vi "Projekt_KSP_main.vi"() -> ()   [LabVIEW 2020]
uses:
  <vilib>/sound2/lvsound2.llb/Sampling Mode.ctl
  <vilib>/sound2/lvsound2.llb/Sound Data Format.ctl
  <vilib>/sound2/lvsound2.llb/Sound Output Set Volume (Single).vi
  <vilib>/Utility/inputDevices.llb/keyboardAcquire.vi
  <vilib>/sound2/lvsound2.llb/Sound Output Write (DBL Single).vi
  <vilib>/Utility/inputDevices.llb/closeKeyboard.vi
  <vilib>/measure/NI_MABase.lvlib
panel:
  in  "Oktawa":dbl min=-3.0 max=4.0 step=1.0
  in  "Amplituda":dbl=1.0
  in  "VOLUME":u32(knob)=100 scale=0.0..100.0
  out "Wykres przebiegu":waveform(dbl)(graph)
  in  "Rodzaj przebiegu":i32
  in  "Podstawa":dbl=261.63
  in  "?":bool
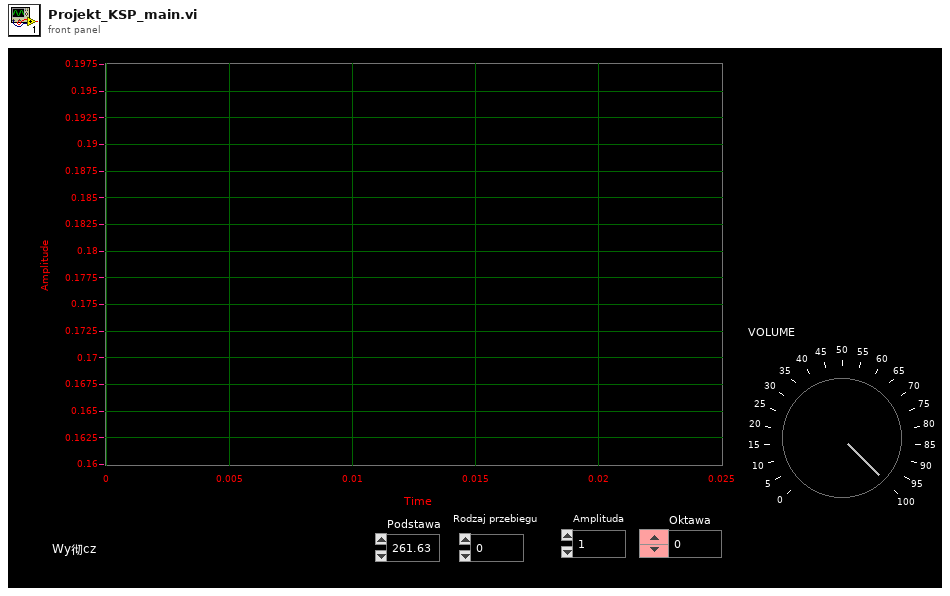
[diagram p1: front panel]
types:
  T1 = typedef "Sound Data Format.ctl" = cluster{"sample rate (S/s)":dbl, "number of channels":i32, "bits per sample":i32}
  T2 = typedef "Sampling Mode.ctl" = i32
  T3 = typedef "Sound Output Task ID.ctl" = u32
  T4 = enum16{"0", "1", "2", "3", "4", "5", "6", "7", "8", "9", "A", "B", "C", "D", "E", "F", "G", "H", "I", "J", "K", "L", "M", "N", "O", "P", "Q", "R", "S", "T", "U", "V", "W", "X", "Y", "Z", "F1", "F2", "F3", "F4", "F5", "F6", "F7", "F8", "F9", "F10", "F11", "F12", "F13", "F14", "F15", "ADD", "BACK", "BACKSLASH", "CAPITAL", "COMMA", "DECIMAL", "DELETE", "DIVIDE", "DOWN", "END", "EQUALS", "ESCAPE", "GRAVE (`)", "HOME", "INSERT", "LBRACKET", "LCONTROL", "LEFT", "L ALT", "LSHIFT", "LWIN", "MINUS", "MULTIPLY", "NEXT", "NUMLOCK", "NUMPAD_0", "NUMPAD_1", "NUMPAD_2", "NUMPAD_3", "NUMPAD_4", "NUMPAD_5", "NUMPAD_6", "NUMPAD_7", "NUMPAD_8", "NUMPAD_9", "PAUSE", "PERIOD", "PRIOR (PG UP)", "RBRACKET", "RCONTROL", "RETURN", "RIGHT", "R ALT", "RSHIFT", "RWIN", "SCROLL", "SEMICOLON", "SLASH", "SPACE", "SUBTRACT", "TAB", "UP", "ENTER (num pad)", "' (quote)"}[]
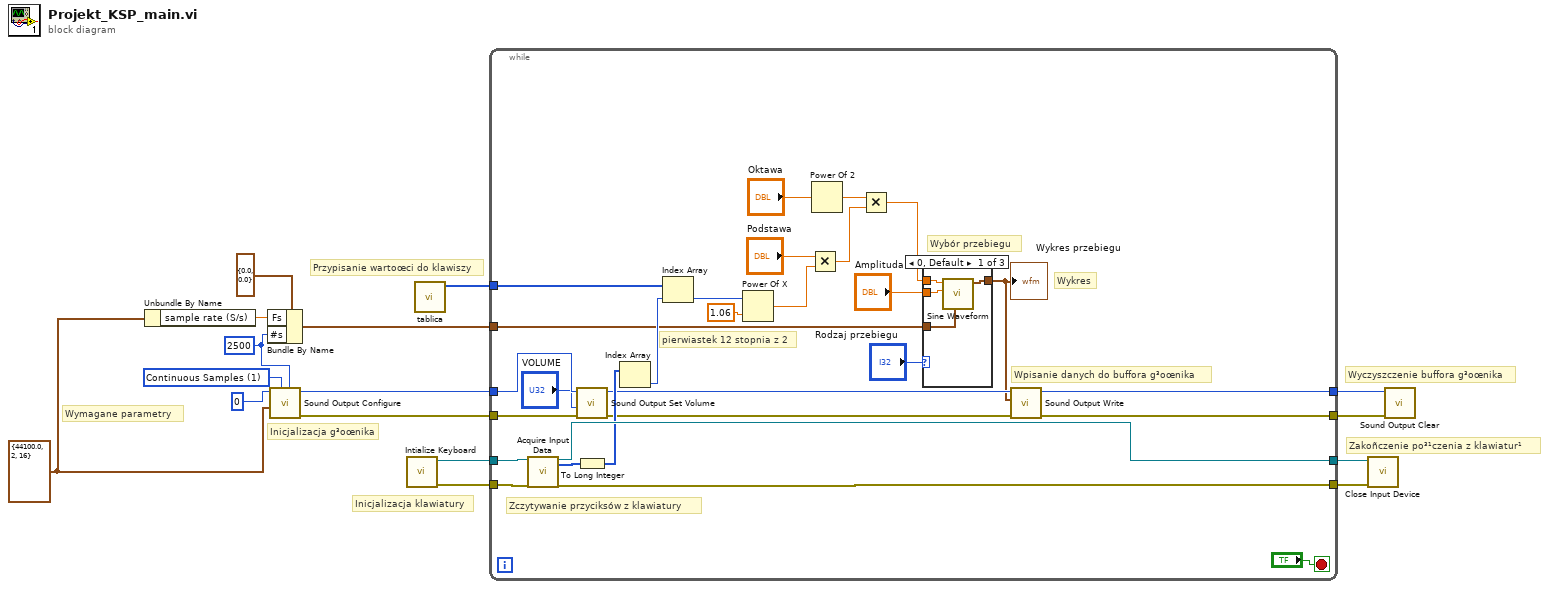
[diagram p0: block diagram]
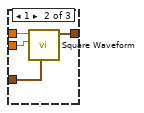
[diagram p2: hidden frame]
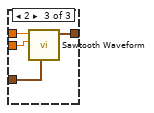
[diagram p3: hidden frame]
diagram:
  w9 = 2500 ("Samples/ch")
  w7 = T1 {"sample rate (S/s)"=44100.0, "number of channels"=2, "bits per sample"=16} ("Sound Format")
  w12 = T2 1 items=["Finite Samples", "Continuous Samples"] ("sample mode")
  # "Wymagane parametry"
  # "Inicjalizacja g³oœnika"
  # "Przypisanie wartoœci do klawiszy"
  # "Wyczyszczenie buffora g³oœnika"
  # "Zakoñczenie po³¹czenia z klawiatur¹"
  # "Inicjalizacja klawiatury"
  n1 = Unbundle By Name(w7) -> ("sample rate (S/s)"=w10:dbl)
  n2 = Bundle By Name(cluster=cluster{"Fs":dbl, "#s":dbl} {"Fs"=0.0, "#s"=0.0} ("sampling info"), "Fs"=w10, "#s"=w9) -> (w6:cluster{"Fs":dbl, "#s":dbl})
  n3 = call <vilib>:"Sound Output Configure.vi"("number of samples/ch"=w9, "sample mode"=w12, "sound format"=w7, "device ID"=u32 0 ("Device ID")) -> ("error out"=w4:errorcluster, "task ID"=w5:T3)  [unwired: 6 in]
  n4 = call <vilib>:"Intialize Keyboard.vi"() -> ("error out"=w16:errorcluster, "device ID"=w13:refnum<k1>)  [unwired: 10 in]
  n5 = call "tablica.vi"() -> ("array"=w1:i32[])  [unwired: 11 in]
  n6 = while {
    tunnel: w13 -> [w43]
    tunnel: w16 -> [w44]
    tunnel: [w41] -> w14
    tunnel: [w42] -> w15
    tunnel: w6 -> [w34]
    tunnel: w5 -> [w29]
    tunnel: [w33] -> w2
    tunnel: [w32] -> w3
    tunnel: w4 -> [w28]
    tunnel: w1 -> [w17]
    stop <- "?" stop-if-true
    # "pierwiastek 12 stopnia z 2"
    # "Wybór przebiegu"
    # "Wykres"
    # "Wpisanie danych do buffora g³oœnika"
    # "Zczytywanie przyciksów z klawiatury"
    n7 = call-poly <vilib>:"Acquire Input Data.vi"("device ID"=w43, "error in (no error)"=w44) -> ("device ID"=w42:refnum<k1>, "keys pressed"=w40:T4, "error out"=w41:errorcluster)  [unwired: 15 in]
    n8 = call-poly <vilib>:"Sound Output Set Volume.vi"("error in (no error)"=w28, "volume"="VOLUME", "task ID"=w29) -> ("error out"=w27:errorcluster, "task ID out"=w30:T3)  [unwired: 7 in]
    n9 = To Long Integer(number=w40) -> (32bit integer=w39:i32[])
    n10 = Index Array(array=w39) -> (element=w38:i32)  [unwired: 1 in]
    n11 = Index Array(array=w17, index=w38) -> (element=w37:i32)
    n12 = Power Of X(1:1.06, 2:w37) -> (0:w25:dbl)
    n13 = Multiply(x="Podstawa", y=w25) -> (x*y=w19:dbl)
    n14 = Power Of 2(x="Oktawa") -> (2^x=w21:dbl)
    n15 = Multiply(x=w21, y=w19) -> (x*y=w18:dbl)
    n16 = case shown="0, Default" "Rodzaj przebiegu" {
      tunnel: w18 -> [w45 w50 w56]
      tunnel: w34 -> [w48 w49 w55]
      tunnel: [w46 w52 w54] -> w24
      tunnel: "Amplituda" -> [w47 w51 w53]
      frame 0, Default {
        n17 = call <vilib>:"Sine Waveform.vi"("sampling info"=w48, "amplitude"=w47, "frequency"=w45) -> ("signal out"=w46:waveform(dbl))  [unwired: 7 in, 1 out]
      }
      frame 1 {
        n18 = call <vilib>:"Square Waveform.vi"("sampling info"=w49, "amplitude"=w51, "frequency"=w50) -> ("signal out"=w52:waveform(dbl))  [unwired: 7 in, 1 out]
      }
      frame 2 {
        n19 = call <vilib>:"Sawtooth Waveform.vi"("sampling info"=w55, "amplitude"=w53, "frequency"=w56) -> ("signal out"=w54:waveform(dbl))  [unwired: 7 in, 1 out]
      }
    }
    "Wykres przebiegu" <- w24
    n20 = call-poly <vilib>:"Sound Output Write.vi"("error in (no error)"=w27, "data"=w24, "task ID"=w30) -> ("error out"=w33:errorcluster, "task ID out"=w32:T3)  [unwired: 7 in]
  }
  n21 = call-poly <vilib>:"Close Input Device.vi"("error in (no error)"=w14, "device ID"=w15) -> ()  [unwired: 8 in, 1 out]
  n22 = call <vilib>:"Sound Output Clear.vi"("error in (no error)"=w2, "task ID"=w3) -> ()  [unwired: 9 in, 1 out]
